vi "load_file_data.vi"(5 "Thermal Coefficient Path":path) -> (2 "Therm Coefs":string[][](array[string]))   [LabVIEW 2010]
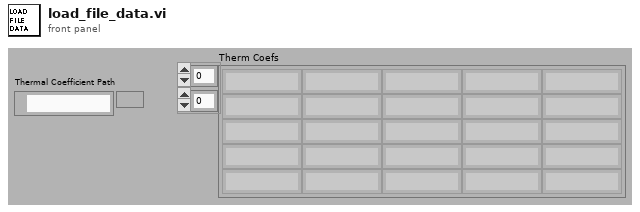
[diagram p1: front panel]
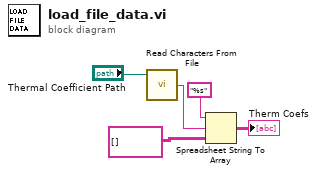
[diagram p0: block diagram]
diagram:
  n1 = call <vilib>:"Read Characters From File.vi"("file path (dialog if empty)"="Thermal Coefficient Path") -> ("character string"=w5:string)  [unwired: 5 in, 3 out]
  n2 = Spreadsheet String To Array(format string="%s", spreadsheet string=w5, array type (2D Dbl)=string[][] [] ("string array")) -> (array=→"Therm Coefs":string[][])  [unwired: 1 in]
